vi "GD_Update_GWID.vi"(8 "error in (no error)":errorcluster, 9 "Next GWID":i32=2, 10 "Current GWID":i32=1, 11 "DBlink":string="Driver={ODBC Driver 17 for SQL Server};Server=localhost\\SQLEXPRESS;Database=ZDX201;UID=labview;PWD=Dsa@54137926") -> (0 "error out":errorcluster)   [LabVIEW 2019]
uses:
  <vilib>/addons/database/Connection.llb/DB Tools Open Connec (String).vi
  <vilib>/addons/database/Connection.llb/Conn Execute.vi
  <vilib>/addons/database/Recordset.llb/Rec Fetch Recordset Data (R).vi
  <vilib>/addons/database/Recordset.llb/Rec Destroy - Connection.vi
  <vilib>/addons/database/_DB Variant To Data/Database Variant To Data.xnode
  <vilib>/addons/database/NI_Database_API.lvlib
panel:
  out "Command 1":string="SELECT TOP (1) [id]      \n FROM [ZDX201].[dbo].[glue_data]\n where glue_workspace_id=1 order by id desc"
  out "Command 2":string="WHERE [id]=13"
  in  "columns":string[](array[string])=["glue_workspace_id", "update_time"]
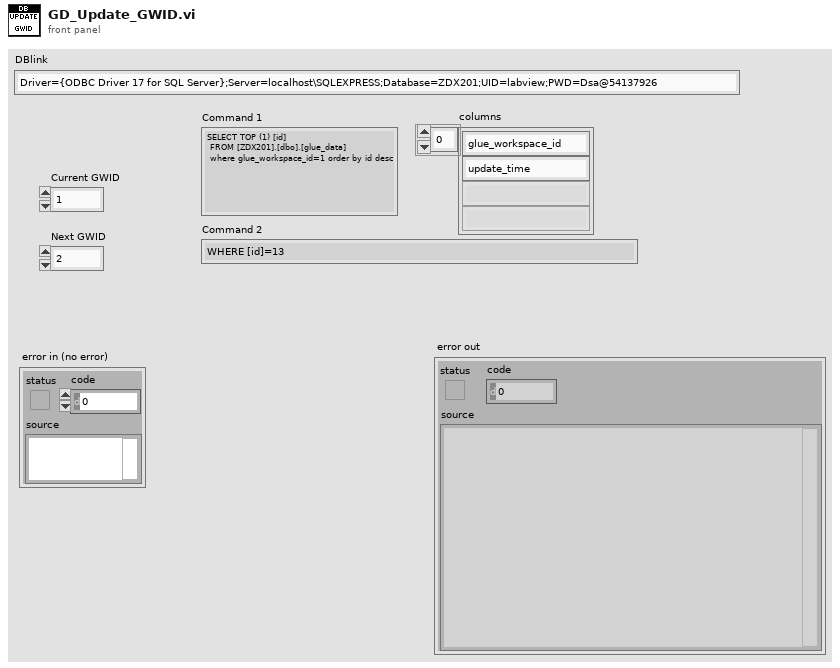
[diagram p1: front panel]
types:
  T1 = cluster{"Next GWID":i32, "update_time":timestamp}
  T2 = typedef "NI_Database_API.lvlib/Conn ObjectReference.ctl" = refnum<k1>
  T3 = typedef "NI_Database_API.lvlib/Rec ObjectReference.ctl" = refnum<k1>
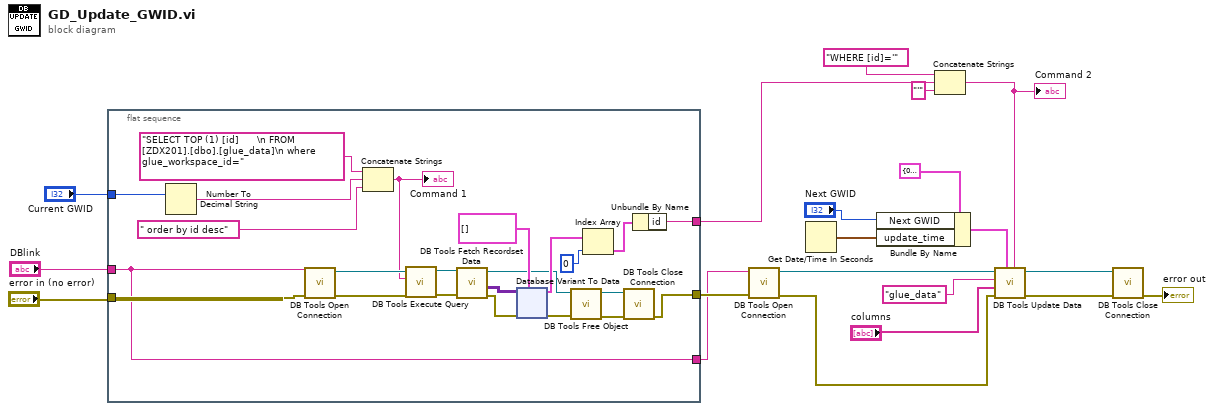
[diagram p0: block diagram]
diagram:
  n1 = flat-sequence {
    tunnel: "DBlink" -> [w24]
    tunnel: "error in (no error)" -> [w43]
    tunnel: "Current GWID" -> [w39]
    tunnel: [w25] -> w4
    tunnel: [w24] -> w3
    tunnel: [w21] -> w2
    frame #0 {
      n2 = Number To Decimal String(number=w39) -> (decimal integer string=w38:string)  [unwired: 1 in]
      n3 = call-poly <vilib>:"DB Tools Open Connection.vi"("error in (no error)"=w43, "connection information"=w24) -> ("error out"=w42:errorcluster, "connection reference"=w41:T2)  [unwired: 6 in]
      n4 = Concatenate Strings("SELECT TOP (1) [id]      \n FROM [ZDX201].[dbo].[glue_data]\n where glue_workspace_id=" ("SQL query"), w38, " order by id desc" ("SQL query")) -> (w36:string)
      "Command 1" <- w36
      n5 = call-poly <vilib>:"DB Tools Execute Query.vi"("error in (no error)"=w42, "SQL query"=w36, "connection reference"=w41) -> ("error out"=w35:errorcluster, "recordset reference"=w34:T3)  [unwired: 5 in]
      n6 = call-poly <vilib>:"DB Tools Fetch Recordset Data.vi"("error in (no error)"=w35, "recordset reference"=w34) -> ("error out"=w33:errorcluster, "recordset data"=w23:variant[][], "recordset reference out"=w26:T3)  [unwired: 3 in]
      n7 = xnode "Database Variant To Data"("database variant"=w23, "error in (no error)"=w33, "type"=cluster{"id":string}[] [] ("initialized array")) -> ("data"=w31:cluster{"id":string}[], "error out"=w27:errorcluster)
      n8 = call-poly <vilib>:"DB Tools Free Object.vi"("error in (no error)"=w27, "recordset reference"=w26) -> ("error out"=w28:errorcluster, "connection reference"=w29:T2)  [unwired: 8 in]
      n9 = Index Array(array=w31, index=0) -> (element=w22:cluster{"id":string})
      n10 = call <vilib>:"DB Tools Close Connection.vi"("error in (no error)"=w28, "connection reference"=w29) -> ("error out"=w25:errorcluster)  [unwired: 5 in]
      n11 = Unbundle By Name(w22) -> ("id"=w21:string)
    }
  }
  n12 = call-poly <vilib>:"DB Tools Open Connection.vi"("error in (no error)"=w4, "connection information"=w3) -> ("error out"=w19:errorcluster, "connection reference"=w8:T2)  [unwired: 6 in]
  n13 = Get Date/Time In Seconds() -> (seconds since 1Jan1904=w11:timestamp)
  n14 = Bundle By Name(cluster=T1 {"Next GWID"=0, "update_time"=timestamp(0 s since 1904-01-01)}, "Next GWID"="Next GWID", "update_time"=w11) -> (w10:T1)
  n15 = Concatenate Strings("WHERE [id]='", w2, "'" ("string")) -> (w13:string)
  "Command 2" <- w13
  n16 = call <vilib>:"DB Tools Update Data.vi"("condition"=w13, "data"=w10, "error in (no error)"=w19, "columns"="columns", "table"="glue_data", "connection reference"=w8) -> ("error out"=w20:errorcluster, "connection reference out"=w18:T2)  [unwired: 4 in]
  n17 = call <vilib>:"DB Tools Close Connection.vi"("error in (no error)"=w20, "connection reference"=w18) -> ("error out"=→"error out":errorcluster)  [unwired: 5 in]
